vi "waitForMagnet.vi"(4 "Type":enum16{"In Range", "Less", "Greater"}(ring), 6 "Axis":T1=enum."Z", 8 "error in (no error)":errorcluster, 9 "Tolerance (T)":dbl, 10 "Setpoint (T)":dbl, 11 "Instrument.Cryostat in":refnum<class "Instrument.Cryostat.lvclass">) -> (0 "error out":errorcluster, 3 "Instrument.Cryostat out":refnum<class "Instrument.Cryostat.lvclass">)   [LabVIEW 2019, in "Instrument.Cryostat.lvclass"]
uses:
  Instrument.Cryostat.lvclass
  Typedefs/Magnet Axis--Enum.ctl
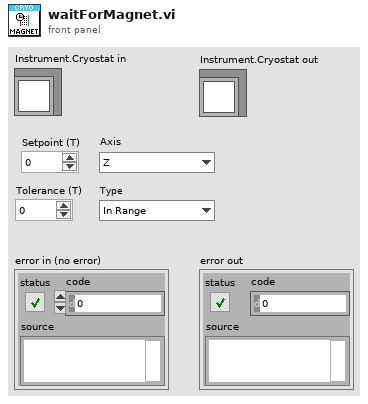
[diagram p1: front panel]
types:
  T1 = typedef "Instrument.Cryostat.lvclass/Magnet Axis--Enum.ctl" = enum16{"X", "Y", "Z"}
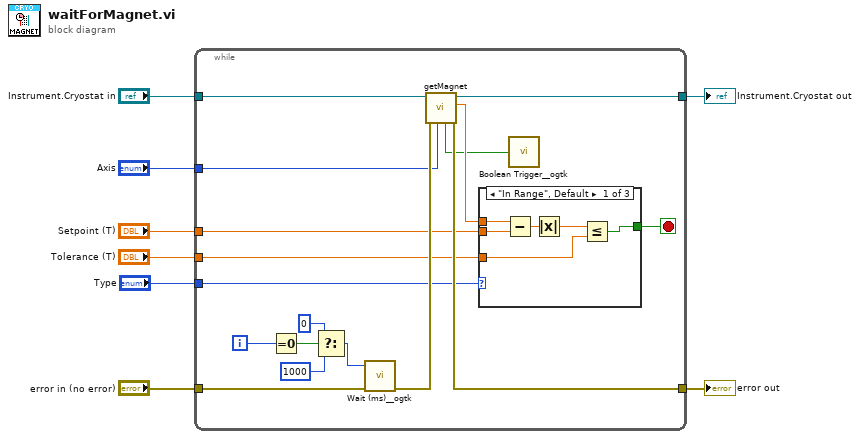
[diagram p0: block diagram]
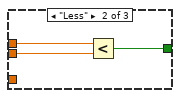
[diagram p2: hidden frame]
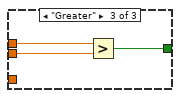
[diagram p3: hidden frame]
diagram:
  n1 = while {
    tunnel: "Setpoint (T)" -> [w12]
    tunnel: "error in (no error)" -> [w23]
    tunnel: [w24] -> w8
    tunnel: "Instrument.Cryostat in" -> [w22]
    tunnel: [w21] -> w4
    tunnel: "Axis" -> [w20]
    tunnel: "Tolerance (T)" -> [w11]
    tunnel: "Type" -> [w10]
    i -> [w19]
    stop <- w14 stop-if-true
    n2 = Equal To 0?(x=w19) -> (x = 0?=w18:bool)
    n3 = Select(t=u32 0, s=w18, f=u32 1000 ("milliseconds to wait")) -> (s? t:f=w15:u32)
    n4 = call <userlib>:"Wait (ms)__ogtk.vi"("error in (no error)"=w23, "milliseconds to wait"=w15) -> ("error out"=w25:errorcluster)  [unwired: 8 in, 1 out]
    n5 = call-dynamic "getMagnet.vi"("Axis"=w20, "error in (no error)"=w25, "Instrument.Cryostat in"=w22) -> ("error out"=w24:errorcluster, "B Field (T)"=w13:dbl, "Instrument.Cryostat out"=w21:refnum<class "Instrument.Cryostat.lvclass">, "Finished?"=w9:bool)  [unwired: 4 in, 1 out]
    n6 = case shown="\"In Range\", Default" w10 {
      tunnel: w12 -> [w29 w34 w37]
      tunnel: [w28 w32 w35] -> w14
      tunnel: w13 -> [w27 w33 w36]
      tunnel: w11 -> [w26 _ _]
      frame "In Range", Default {
        n7 = Subtract(x=w27, y=w29) -> (x-y=w31:dbl)
        n8 = Absolute Value(x=w31) -> (abs(x)=w30:dbl)
        n9 = Less Or Equal?(x=w30, y=w26) -> (x <= y?=w28:bool)
      }
      frame "Less" {
        n10 = Less?(x=w33, y=w34) -> (x < y?=w32:bool)
      }
      frame "Greater" {
        n11 = Greater?(x=w36, y=w37) -> (0:w35:bool)
      }
    }
    n12 = call <userlib>:"Boolean Trigger__ogtk.vi"("Boolean Input"=w9) -> ()  [unwired: 1 in, 2 out]
  }
  "Instrument.Cryostat out" <- w4
  "error out" <- w8
